vi "FTW-SEQ-AddNext.vi"(1 "Add Next in Sequence":string, 3 "FTW Job Sequencer":refnum<class "FTW-JobSequencer.lvclass">) -> (0 "FTW Job Sequencer out":refnum<class "FTW-JobSequencer.lvclass">)   [LabVIEW 2012, in "FTW-Actor.lvlib" / "FTW-JobSequencer.lvclass"]
uses:
  FTW-JobSequencer.lvclass
  FTW-JobSequencer.lvclass/FTW-JobSequencer.ctl
panel:
  # "Inputs"
  # "Outputs"
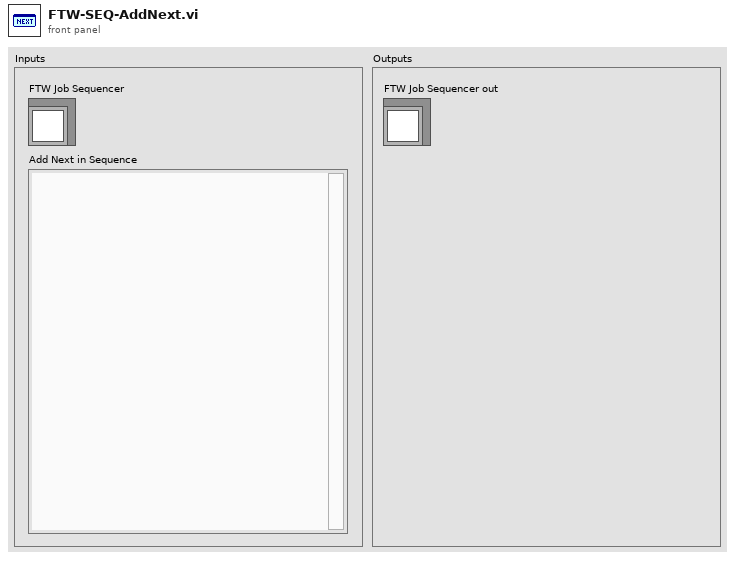
[diagram p1: front panel]
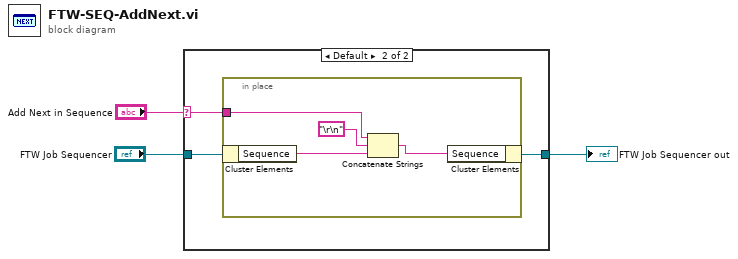
[diagram p0: block diagram]
diagram:
  n1 = case shown="Default" "Add Next in Sequence" {
    selector: "Add Next in Sequence" -> [_ w5]
    tunnel: "FTW Job Sequencer" -> [w4 w7]
    tunnel: [w4 w6] -> w2
    frame "" {
    }
    frame Default {
      n2 = in-place {
        in-place-border: w5 -> [w8]
        n3 = in-place-cluster #1(w7) -> ("Sequence"=w11:string)
        n4 = Concatenate Strings(w8, "\r\n", w11) -> (w9:string)
        n5 = in-place-cluster #1("Sequence"=w9) -> (w6:refnum<class "FTW-JobSequencer.lvclass">)
      }
    }
  }
  "FTW Job Sequencer out" <- w2
